vi "Test Create Table.vi"(6 "Additional constraints":string[](array[string]), 8 "error in (no error)":errorcluster, 9 "Columns Type Affinity":enum16{"TEXT", "NUM", "INT", "REAL", "BLOB"}[](array[ring]), 10 "Column Names":string[](array[string]), 11 "database in":path) -> (0 "error out":errorcluster, 1 "PRAGMA table info":string[][](array[string]))   [LabVIEW 2020, in "sqlite3.lvlib"]
uses:
  sqlite3.lvlib
  <vilib>/Utility/error.llb/Clear Errors.vi
  sqlite/VIs/open v2.vi
  sqlite/VIs/prepare v2.vi
  sqlite/VIs/step.vi
  sqlite/VIs/column count.vi
  compound/Column.vi
  compound/Resolve Result Type.vi
  sqlite/VIs/finalize.vi
  sqlite/VIs/close v2.vi
  sqlite/subvi/Error Converter (ErrCode or Status).vi
  sqlite/VIs/column text.vi
  sqlite/VIs/column bytes.vi
  sqlite/VIs/column blob.vi
  utilities/MoveBlock.vi
  sqlite/VIs/column type.vi
  sqlite/VIs/errstr.vi
panel:
  out "created?":bool
  in  "Table name in":string
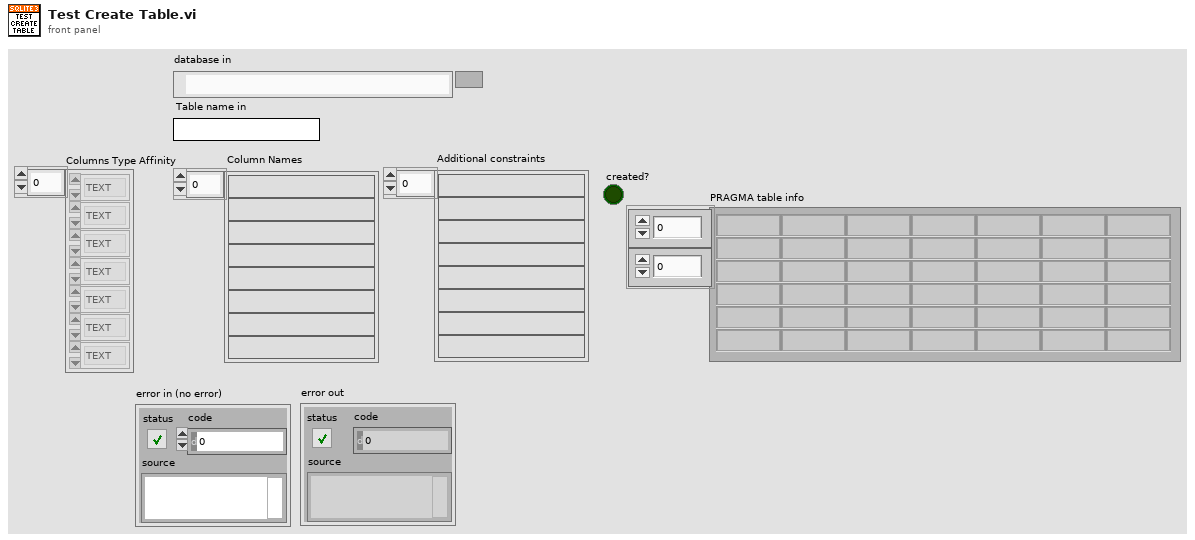
[diagram p1: front panel]
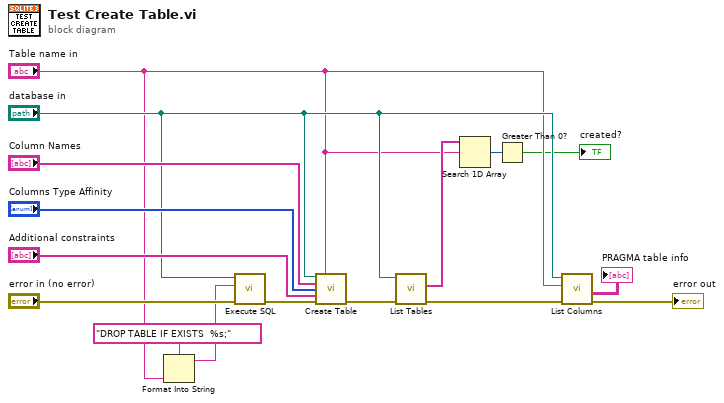
[diagram p0: block diagram]
diagram:
  n1 = Format Into String(format string="DROP TABLE IF EXISTS  %s;" ("sql (string)"), "Table name in") -> (resulting string=w8:string)  [unwired: 2 in, 1 out]
  n2 = call "Execute SQL.vi"("error in (no error)"="error in (no error)", "sql (string)"=w8, "database in"="database in") -> ("error out"=w10:errorcluster)  [unwired: 7 in, 1 out]
  n3 = call "Create Table.vi"("database in"="database in", "Table name in"="Table name in", "Column Names"="Column Names", "Columns Type Affinity"="Columns Type Affinity", "Additional constraints"="Additional constraints", "error in (no error)"=w10) -> ("error out"=w12:errorcluster)  [unwired: 9 in]
  n4 = call "List Tables.vi"("error in (no error)"=w12, "database in"="database in") -> ("error out"=w6:errorcluster, "Tables"=w13:string[])  [unwired: 8 in]
  n5 = Search 1D Array(1D array=w13, element="Table name in") -> (index of element=w7:i32)  [unwired: 1 in]
  n6 = Greater Than 0?(x=w7) -> (x > 0?=→"created?":bool)
  n7 = call "List Columns.vi"("error in (no error)"=w6, "Table name"="Table name in", "database in"="database in") -> ("error out"=→"error out":errorcluster, "PRAGMA table info"=→"PRAGMA table info":string[][])  [unwired: 5 in, 2 out]
